vi "Exposure-Init Stimulus.vi"(0 "Exposure parameters":T24, 1 "Data Folder":path, 7 "Sampling rate (Hz)":dbl, 9 "Npts":i32, 11 "error in (no error)":errorcluster, 12 "Seeds":cluster{"Left":i32, "Right":i32}, 13 "Filter options":cluster{"InvFilt":bool, "Brickwall":bool}) -> (4 "StimChan":T23(array[cluster]) {"Filter"."IIR Filter Cluster"."Forward Coefficients" format="%.4f"; "Filter"."IIR Filter Cluster"."Reverse Coefficients" format="%.4f"}, 6 "InvFilt":T1[](array[typedef]), 14 "Max Level":dbl[](array[numeric]), 15 "error out":errorcluster)   [LabVIEW 2020]
uses:
  Typedefs/Exposure Parameters.ctl
  epl-vi-lib/Signal Synthesis VIs/Controls/Waveform XCtl/Waveform Data.ctl
  epl-vi-lib/Signal Synthesis VIs/Controls/Waveform XCtl/Waveform Enum.ctl
  epl-vi-lib/Signal Synthesis VIs/Waveform VIs/Tone VIs/Tone Params.ctl
  epl-vi-lib/Signal Synthesis VIs/Waveform VIs/Pulse Train VIs/Pulse Train Params.ctl
  epl-vi-lib/Signal Synthesis VIs/Waveform VIs/Pulse Train VIs/Pulse Polarity.ctl
  epl-vi-lib/Signal Synthesis VIs/Waveform VIs/Pulse Train VIs/PT-Continuous State.ctl
  epl-vi-lib/Signal Synthesis VIs/Waveform VIs/Noise VIs/Noise Params.ctl
  epl-vi-lib/Signal Synthesis VIs/Waveform VIs/File VIs/StimFile-Params.ctl
  epl-vi-lib/Signal Synthesis VIs/Waveform VIs/FM Sweep VIs/FM Sweep Params.ctl
  epl-vi-lib/Signal Synthesis VIs/Waveform VIs/Chirp Train VIs/Chirp Train.ctl
  epl-vi-lib/Signal Synthesis VIs/Waveform VIs/Chirp Train VIs/Chirp Train Params.ctl
  epl-vi-lib/Signal Synthesis VIs/Waveform VIs/Complex Tone VIs/CT-Params.ctl
  epl-vi-lib/Signal Synthesis VIs/Waveform VIs/Complex Tone VIs/CT-Phase Enum.ctl
  epl-vi-lib/Signal Synthesis VIs/Waveform VIs/Complex Tone VIs/CT-Runtime Data.ctl
  epl-vi-lib/Signal Synthesis VIs/Waveform VIs/Moving Ripple VIs/Moving Ripple.ctl
  epl-vi-lib/Signal Synthesis VIs/Waveform VIs/Moving Ripple VIs/Moving Ripple.Params.ctl
  epl-vi-lib/Signal Synthesis VIs/Waveform VIs/Moving Ripple VIs/Moving Ripple.Data.ctl
  epl-vi-lib/Signal Synthesis VIs/Controls/Filter XCtl/Filter Data.ctl
  epl-vi-lib/Signal Synthesis VIs/Controls/Gate XCtl/Gate Data.ctl
  epl-vi-lib/Signal Synthesis VIs/Controls/Level XCtl/Level Data.ctl
  epl-vi-lib/Signal Synthesis VIs/Controls/Level XCtl/Level Units.ctl
  Typedefs/Exposure-Inverse Filter Runtime.ctl
  epl-cal-vi-lib/Inverse Filter VIs/InvFilt-Params.ctl
  epl-vi-lib/Utility VIs/Type Defs/Speaker ring.ctl
  epl-vi-lib/Signal Synthesis VIs/Controls/Level XCtl/Level XCtl.xctl
  epl-vi-lib/Signal Synthesis VIs/Controls/Gate XCtl/Gate Control.xctl
  epl-vi-lib/Signal Synthesis VIs/Controls/Filter XCtl/Filter XCtl.xctl
  epl-vi-lib/Signal Synthesis VIs/Controls/Waveform XCtl/Waveform XCtl.xctl
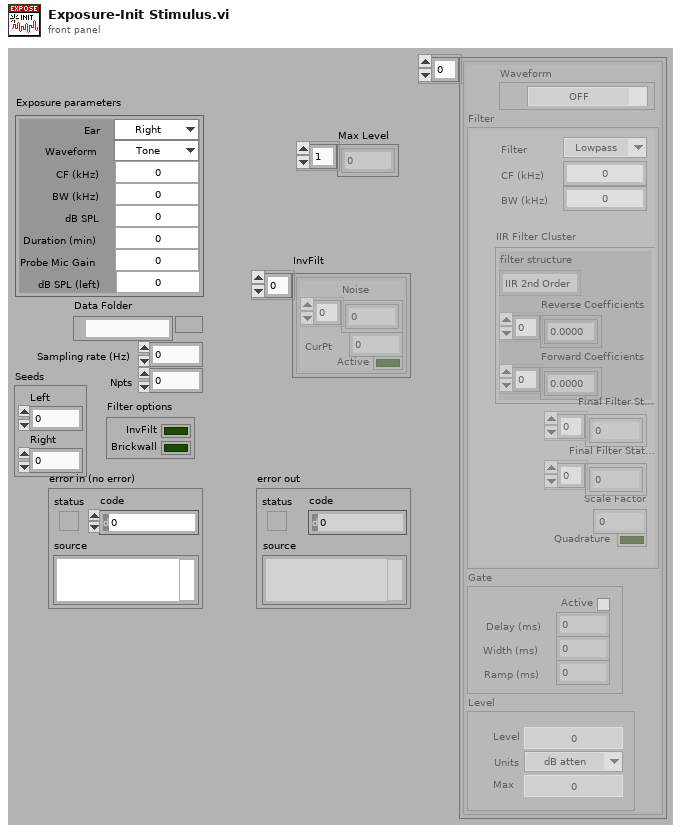
[diagram p1: front panel]
types:
  T1 = typedef "Exposure-Inverse Filter Runtime.ctl" = cluster{"Noise":dbl[], "CurPt":i32, "Active":bool}
  T2 = typedef "Waveform XCtl.xctl/Waveform Data.ctl" = cluster{"Type":T3, "Tone":T4, "Pulse Train":T5, "Noise":T8, "File":T9, "FMSweep":T10, "Chirp Train":T11, "Complex Tone":cluster{"Params":T13, "Data":T15}, "Moving Ripple":T16}
  T3 = typedef "Waveform Enum.ctl" = enum16{"OFF", "Tone", "Noise", "Pulse Train", "File", "FM Sweep", "Chirp Train", "Complex Tone", "FM Tone", "Moving Ripple"}
  T4 = typedef "Tone Params.ctl" = cluster{"Frequency (kHz)":dbl, "Last Freq":dbl, "Last Phase":dbl}
  T5 = typedef "Pulse Train Params.ctl" = cluster{"Pulse width (us)":dbl, "Pulse rate (Hz)":dbl, "Gap (ms)":dbl, "Polarity":T6, "PT State":T7, "Asynch":bool}
  T6 = typedef "Pulse Polarity.ctl" = enum16{"POS", "NEG", "POS-NEG", "NEG-POS"}
  T7 = typedef "PT-Continuous State.ctl" = cluster{"Template":dbl[], "Nperiod":i32, "Index":i32, "Pulse Rate (Hz)":dbl, "Phase (cycles)":dbl, "Noff":i32}
  T8 = typedef "Noise Params.ctl" = cluster{"InvFilt":bool, "Noise":dbl[], "CurPt":i32, "Aweight":bool, "Seed":i32, "afile":path}
  T9 = typedef "StimFile-Params.ctl" = cluster{"Filename":path, "Signal":dbl[], "Channel":i32, "stream":bool, "offset":i32, "nreps":i32, "loops":i32, "Randomize":bool, "order":i32[], "Seed":i32, "Tokens":i32}
  T10 = typedef "FM Sweep Params.ctl" = cluster{"Rate (oct/s)":dbl, "Fmin (Hz)":dbl, "Fmax (Hz)":dbl, "Ramp (ms)":dbl, "Linear":bool}
  T11 = typedef "Chirp Train.ctl" = cluster{"Params":T12, "Data":cluster{"WF":dbl[]}}
  T12 = typedef "Chirp Train Params.ctl" = cluster{"Fmin (kHz)":dbl, "Fmax (kHz)":dbl, "Compensate":bool, "Duration (ms)":dbl}
  T13 = typedef "CT-Params.ctl" = cluster{"F0 (Hz)":dbl, "Band":cluster{"Flow (Hz)":dbl, "Fhigh (Hz)":dbl}, "Phase":T14, "Min F0 (Hz)":dbl, "Max F0 (Hz)":dbl, "ContinRandPhase":bool, "Max peak factor":dbl, "Max mod depth":dbl, "MinHarmNum":i32, "MaxHarmNum":i32, "Level Mode":enum16{"per component", "overall rms"}, "% jitter":dbl}
  T14 = typedef "CT-Phase Enum.ctl" = enum16{"Cosine", "Random", "Alternating"}
  T15 = typedef "CT-Runtime Data.ctl" = cluster{"Ncomp":i32, "MinHarm":i32, "Phase":dbl[], "Amplitude":dbl[], "Npts/frame":i32, "Last F0":dbl, "Fmin":dbl, "Fmax":dbl, "Lslope":dbl, "randphase":bool, "overall rms":bool, "fmult":dbl[], "jittered":bool}
  T16 = typedef "Moving Ripple.ctl" = cluster{"Params":T17, "Data":T18}
  T17 = typedef "Moving Ripple.Params.ctl" = cluster{"Fmin":dbl, "Fmax":dbl, "Density":dbl, "Velocity":dbl, "Depth":dbl, "Phase":dbl, "Comp/oct":i32}
  T18 = typedef "Moving Ripple.Data.ctl" = cluster{"Freq":dbl[], "A":dbl[], "phase":dbl[], "Phase":dbl}
  T19 = typedef "Filter XCtl.xctl/Filter Data.ctl" = cluster{"CF (kHz)":dbl, "BW (kHz)":dbl, "IIR Filter Cluster":cluster{"filter structure":enum32{"IIR 2nd Order", "IIR 4th Order"}, "Reverse Coefficients":dbl[], "Forward Coefficients":dbl[]}, "Final Filter State":dbl[], "Scale Factor":dbl, "Final Filter State 2":dbl[], "Quadrature":bool, "Type":enum16{"Lowpass", "Highpass", "Bandpass", "Bandstop", "OFF"}}
  T20 = typedef "Gate Control.xctl/Gate Data.ctl" = cluster{"Active":bool, "Delay (ms)":dbl, "Width (ms)":dbl, "Ramp (ms)":dbl}
  T21 = typedef "Level XCtl.xctl/Level Data.ctl" = cluster{"Level":dbl, "Units":T22, "Max":dbl, "Multiplier":dbl, "Cal File":path, "Cal":cluster{"Freq (Hz)":dbl[], "Mag (dB SPL)":dbl[], "Phase (deg)":dbl[]}}
  T22 = typedef "Level Units.ctl" = enum16{"dB atten", "dB SPL", "dB re 1 Vrms", "dB V/Hz½", "mW", "dB HL", "Volts", "dB mW"}
  T23 = cluster{"Waveform":T2, "Filter":T19, "Gate":T20, "Level":T21}[]
  T24 = typedef "Exposure Parameters.ctl" = cluster{"Probe Mic Gain":dbl, "Waveform":enum16{"Tone", "Noise"}, "CF (kHz)":dbl, "BW (kHz)":dbl, "Ear":enum16{"Right", "Left", "Binaural"}, "Duration (min)":dbl, "dB SPL":dbl, "dB SPL (left)":dbl}
  T25 = cluster{"Waveform":T2, "Filter":T19, "Gate":T20, "Level":T21}
  T26 = typedef "Speaker ring.ctl" = enum16{"Right primary", "Right secondary", "Left primary", "Left secondary"}
  T27 = typedef "InvFilt-Params.ctl" = cluster{"Min Frequency (Hz)":dbl, "Max Frequency (Hz)":dbl, "Length (points)":i32, "Sampling rate (Hz)":dbl, "Delay (ms)":dbl, "Linear phase":bool}
  T28 = enum16{"Lowpass", "Highpass", "Bandpass", "Bandstop", "OFF"}
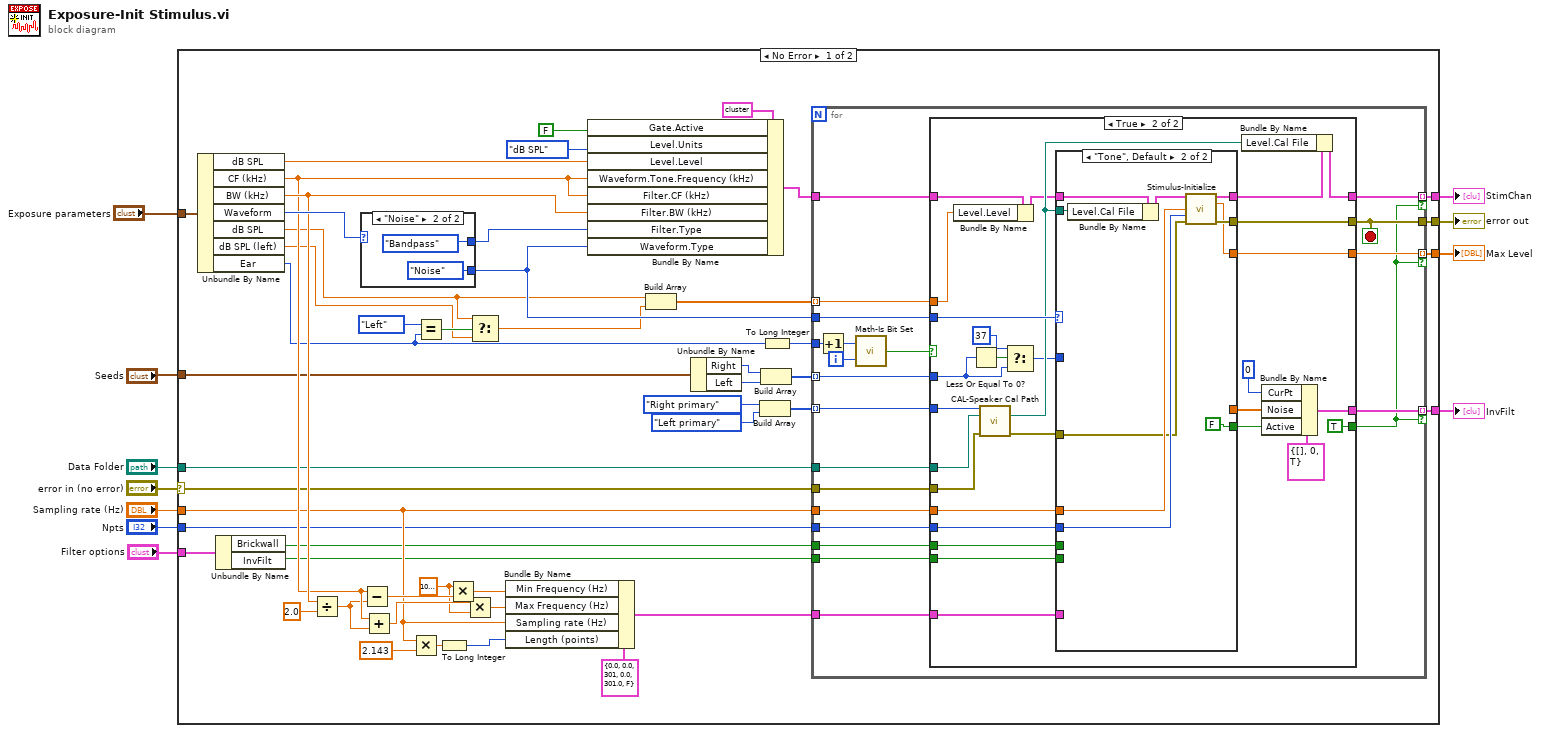
[diagram p0: block diagram]
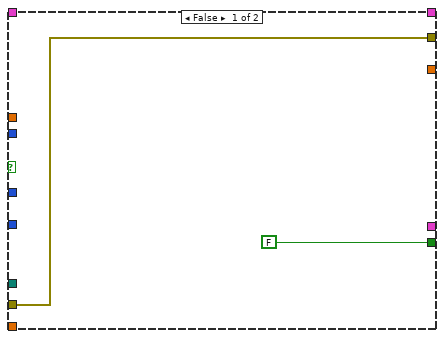
[diagram p2: hidden frame]
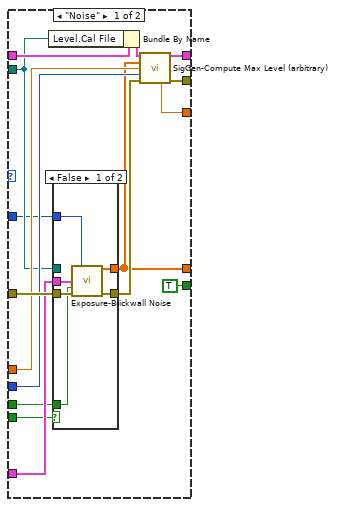
[diagram p3: hidden frame]
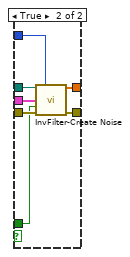
[diagram p4: hidden frame]
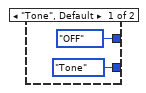
[diagram p5: hidden frame]
diagram:
  n1 = case shown="No Error" "error in (no error)" {
    selector: "error in (no error)" -> [w31 w154]
    tunnel: "Exposure parameters" -> [w59 _]
    tunnel: [w43 w154] -> w10
    tunnel: [w42 _] -> w9
    tunnel: [w38 _] -> w8
    tunnel: "Sampling rate (Hz)" -> [w37 _]
    tunnel: "Npts" -> [w36 _]
    tunnel: [w32 _] -> w5
    tunnel: "Data Folder" -> [w30 _]
    tunnel: "Filter options" -> [w25 _]
    tunnel: "Seeds" -> [w22 _]
    frame No Error {
      w39 = 1000.0 ("x")
      n2 = Unbundle By Name(w59) -> ("dB SPL"=w58:dbl, "CF (kHz)"=w50:dbl, "BW (kHz)"=w53:dbl, "Waveform"=w60:enum16{"Tone", "Noise"}, "dB SPL"=w14:dbl, "dB SPL (left)"=w13:dbl, "Ear"=w17:enum16{"Right", "Left", "Binaural"})
      n3 = Unbundle By Name(w25) -> ("Brickwall"=w23:bool, "InvFilt"=w24:bool)
      n4 = Divide(x=w53, y=2.0) -> (x/y=w49:dbl)
      n5 = case shown="\"Noise\"" w60 {
        tunnel: [T28."OFF" ("Filter.Type") T28."Bandpass" ("Filter.Type")] -> w55
        tunnel: [Waveform_Enum."Tone" ("Waveform.Type") Waveform_Enum."Noise" ("Waveform.Type")] -> w34
        frame "Tone", Default {
        }
        frame "Noise" {
        }
      }
      n6 = Subtract(x=w50, y=w49) -> (x-y=w51:dbl)
      n7 = Add(x=w50, y=w49) -> (x+y=w48:dbl)
      n8 = Multiply(x=w37, y=2.143) -> (x*y=w46:dbl)
      n9 = Equal?(x=enum16{"Right", "Left", "Binaural"}."Left", y=w17) -> (x = y?=w15:bool)
      n10 = To Long Integer(number=w46) -> (32bit integer=w45:i32)
      n11 = Multiply(x=w39, y=w51) -> (x*y=w41:dbl)
      n12 = Multiply(x=w48, y=w39) -> (x*y=w40:dbl)
      n13 = Select(t=w14, s=w15, f=w13) -> (s? t:f=w12:dbl)
      n14 = Bundle By Name(cluster=T27 {"Min Frequency (Hz)"=0.0, "Max Frequency (Hz)"=0.0, "Length (points)"=301, "Sampling rate (Hz)"=0.0, "Delay (ms)"=301.0, "Linear phase"=FALSE} ("InvFilt Params"), "Min Frequency (Hz)"=w41, "Max Frequency (Hz)"=w40, "Sampling rate (Hz)"=w37, "Length (points)"=w45) -> (w44:T27)
      n15 = Bundle By Name(cluster=T25 {"Waveform"={"Type"=enum."Tone", "Tone"={"Frequency (kHz)"=1.0, "Last Freq"=0.0, "Last Phase"=0.0}, "Pulse Train"={"Pulse width (us)"=0.0, "Pulse rate (Hz)"=0.0, "Gap (ms)"=0.0, "Polarity"=enum."POS", "PT State"={"Template"=[], "Nperiod"=0, "Index"=0, "Pulse Rate (Hz)"=0.0, "Phase (cycles)"=0.0, "Noff"=0}, "Asynch"=FALSE}, "Noise"={"InvFilt"=FALSE, "Noise"=[], "CurPt"=0, "Aweight"=FALSE, "Seed"=0, "afile"=path ""}, "File"={"Filename"=path "", "Signal"=[], "Channel"=0, "stream"=FALSE, "offset"=0, "nreps"=0, "loops"=0, "Randomize"=FALSE, "order"=[], "Seed"=0, "Tokens"=0}, "FMSweep"={"Rate (oct/s)"=0.0, "Fmin (Hz)"=0.0, "Fmax (Hz)"=0.0, "Ramp (ms)"=0.0, "Linear"=FALSE}, "Chirp Train"={"Params"={"Fmin (kHz)"=0.0, "Fmax (kHz)"=0.0, "Compensate"=FALSE, "Duration (ms)"=0.0}, "Data"={"WF"=[]}}, "Complex Tone"={"Params"={"F0 (Hz)"=0.0, "Band"={"Flow (Hz)"=0.0, "Fhigh (Hz)"=0.0}, "Phase"=enum."Cosine", "Min F0 (Hz)"=0.0, "Max F0 (Hz)"=0.0, "ContinRandPhase"=FALSE, "Max peak factor"=0.0, "Max mod depth"=0.0, "MinHarmNum"=0, "MaxHarmNum"=0, "Level Mode"=enum."per component", "% jitter"=0.0}, "Data"={"Ncomp"=0, "MinHarm"=0, "Phase"=[], "Amplitude"=[], "Npts/frame"=0, "Last F0"=0.0, "Fmin"=0.0, "Fmax"=0.0, "Lslope"=0.0, "randphase"=FALSE, "overall rms"=FALSE, "fmult"=[], "jittered"=FALSE}}, "Moving Ripple"={"Params"={"Fmin"=0.0, "Fmax"=0.0, "Density"=0.0, "Velocity"=0.0, "Depth"=0.0, "Phase"=0.0, "Comp/oct"=0}, "Data"={"Freq"=[], "A"=[], "phase"=[], "Phase"=0.0}}}, "Filter"={"CF (kHz)"=1.0, "BW (kHz)"=4.0, "IIR Filter Cluster"={"filter structure"=enum."IIR 2nd Order", "Reverse Coefficients"=[], "Forward Coefficients"=[]}, "Final Filter State"=[], "Scale Factor"=0.0, "Final Filter State 2"=[], "Quadrature"=FALSE, "Type"=enum."OFF"}, "Gate"={"Active"=FALSE, "Delay (ms)"=0.0, "Width (ms)"=0.0, "Ramp (ms)"=0.0}, "Level"={"Level"=120.0, "Units"=enum."dB SPL", "Max"=nan, "Multiplier"=0.0, "Cal File"=path "/RightPrimary.calib", "Cal"={"Freq (Hz)"=[], "Mag (dB SPL)"=[], "Phase (deg)"=[]}}} ("StimChan"), "Gate.Active"=FALSE, "Level.Units"=Level_Units."dB SPL" ("Level.Mode"), "Level.Level"=w58, "Waveform.Tone.Frequency (kHz)"=w50, "Filter.CF (kHz)"=w50, "Filter.BW (kHz)"=w53, "Filter.Type"=w55, "Waveform.Type"=w34) -> (w35:T25)
      n16 = Build Array(w14, w12) -> (w18:dbl[])
      n17 = Unbundle By Name(w22) -> ("Right"=w21:i32, "Left"=w20:i32)
      n18 = Build Array(Speaker_ring."Right primary" ("Speaker"), Speaker_ring."Left primary" ("Speaker")) -> (w27:T26[])
      n19 = Build Array(w21, w20) -> (w19:i32[])
      n20 = To Long Integer(number=w17) -> (32bit integer=w26:i32)
      n21 = for {
        tunnel: w44 -> [w81]
        tunnel: [w72] -> w43
        tunnel: [w80] -> w42 mode=indexing if=w69
        tunnel: [w73] -> w32 mode=indexing if=w69
        tunnel: [w79] -> w38 mode=indexing if=w69
        tunnel: w37 -> [w78]
        tunnel: w36 -> [w77]
        tunnel: w35 -> [w76]
        tunnel: w31 -> [w68]
        tunnel: w34 -> [w75]
        tunnel: w24 -> [w74]
        tunnel: w26 -> [w70]
        tunnel: w30 -> [w67]
        tunnel: w27 -> [w65] mode=indexing
        tunnel: w23 -> [w63]
        tunnel: w19 -> [w62] mode=indexing
        tunnel: w18 -> [w61] mode=indexing
        i -> [w71]
        stop <- w72 stop-if-true
        n22 = Increment(x=w70) -> (x+1=w64:i32)
        n23 = call "Math-Is Bit Set.vi"("Bit"=w71, "Integer"=w64) -> ("Is Bit Set?"=w66:bool)
        n24 = case shown="True" w66 {
          tunnel: w81 -> [_ w111]
          tunnel: [_ w110] -> w80
          tunnel: [_ w107] -> w79
          tunnel: w78 -> [_ w106]
          tunnel: w77 -> [_ w105]
          tunnel: w76 -> [_ w91]
          tunnel: w75 -> [_ w104]
          tunnel: w74 -> [_ w103]
          tunnel: [_ w100] -> w73
          tunnel: [w82 w99] -> w72
          tunnel: w65 -> [_ w97]
          tunnel: [FALSE TRUE] -> w69
          tunnel: w68 -> [w82 w96]
          tunnel: w67 -> [_ w94]
          tunnel: w63 -> [_ w92]
          tunnel: w62 -> [_ w88]
          tunnel: w61 -> [_ w84]
          frame False {
          }
          frame True {
            n25 = Bundle By Name(cluster=w91, "Level.Level"=w84) -> (w85:T25)
            n26 = Less Or Equal To 0?(x=w88) -> (x <= 0?=w89:bool)
            n27 = call "CAL-Speaker Cal Path.vi"("Speaker"=w97, "Data Folder"=w94, "error in (no error)"=w96) -> ("Cal Path"=w93:path, "error out"=w98:errorcluster)  [unwired: 11 in]
            n28 = Select(t=37, s=w89, f=w88) -> (s? t:f=w86:i32)
            n29 = case shown="\"Tone\", Default" w104 {
              tunnel: w98 -> [w126 w145]
              tunnel: w93 -> [w114 w140]
              tunnel: [w118 _] -> w90
              tunnel: w111 -> [w125 _]
              tunnel: [w124 w144] -> w99
              tunnel: w85 -> [w123 w149]
              tunnel: [w122 w148] -> w108
              tunnel: [w121 w143] -> w107
              tunnel: w106 -> [w120 w147]
              tunnel: w105 -> [w119 w146]
              tunnel: w103 -> [w117 _]
              tunnel: [TRUE FALSE] -> w102
              tunnel: w92 -> [w113 _]
              tunnel: w86 -> [w112 _]
              frame "Noise" {
                n30 = Bundle By Name(cluster=w123, "Level.Cal File"=w114) -> (w115:T25)
                n31 = case shown="False" w117 {
                  tunnel: w126 -> [w132 w139]
                  tunnel: w114 -> [_ w138]
                  tunnel: w125 -> [w129 w137]
                  tunnel: [w131 w136] -> w124
                  tunnel: [w130 w135] -> w118
                  tunnel: w113 -> [w128 w134]
                  tunnel: w112 -> [w127 w133]
                  frame False {
                    n32 = call "Exposure-Brickwall Noise.vi"("seed"=w127, "InvFilt Params"=w129, "Brickwall (T)"=w128, "error in (no error)"=w132) -> ("Noise"=w130:dbl[], "error out"=w131:errorcluster)  [unwired: 9 in, 1 out]
                  }
                  frame True {
                    n33 = call "InvFilter-Create Noise.vi"("Calibration File"=w138, "seed"=w133, "InvFilt Params"=w137, "Brickwall (T)"=w134, "error in (no error)"=w139) -> ("InvFilter Noise"=w135:dbl[], "error out"=w136:errorcluster)  [unwired: 7 in, 2 out]
                  }
                }
                n34 = call "SigGen-Compute Max Level (arbitrary).vi"("Stimulus Channel"=w115, "Y"=w118, "Sampling Rate (Hz)"=w120, "Npts"=w119) -> ("Stimulus Channel out"=w122:T25, "Max Level"=w121:dbl)  [unwired: 9 in, 1 out]
              }
              frame "Tone", Default {
                n35 = Bundle By Name(cluster=w149, "Level.Cal File"=w140) -> (w141:T25)
                n36 = call "Stimulus-Initialize.vi"("Stimulus Channel"=w141, "Sampling rate (Hz)"=w147, "Npts"=w146, "error in (no error)"=w145) -> ("Stimulus Channel out"=w148:T25, "Max Level"=w143:dbl, "error out"=w144:errorcluster)  [unwired: 9 in]
              }
            }
            n37 = Bundle By Name(cluster=w108, "Level.Cal File"=w93) -> (w100:T25)
            n38 = Bundle By Name(cluster=T1 {"Noise"=[], "CurPt"=0, "Active"=TRUE} ("InvFilt 2"), "CurPt"=0, "Noise"=w90, "Active"=w102) -> (w110:T1)
          }
        }
      }
    }
    frame Error {
    }
  }
  "error out" <- w10
  "StimChan" <- w5
  "InvFilt" <- w9
  "Max Level" <- w8
